vi "Set DDC Mode.vi"(0 "fpga refnum":refnum<k20>, 5 "DDC Enabled":bool, 7 "IQ Enabled":bool, 9 "DDC Frequency Shift (Hz)":dbl, 11 "error in (no error)":errorcluster) -> (4 "fpga refnum out":refnum<k20>, 8 "sample rate":dbl, 15 "error out":errorcluster)   [LabVIEW 2018, in "GettingStarted_5785_Host.lvlib"]
uses:
  GettingStarted_5785_Host.lvlib
  <instrlib>/FlexRIO/API/Host/v1/NI FlexRIO/API/Get Property Reference - Fpga Small.vi
  <resource>/objmgr/niflexrioapiStream.rc
  <instrlib>/FlexRIO/API/Host/v1/NI FlexRIO API v1.lvlib
  <resource>/objmgr/niflexrioapiChannel.rc
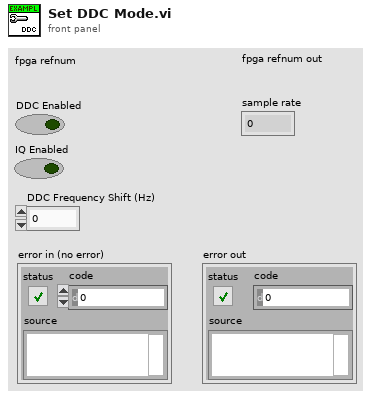
[diagram p1: front panel]
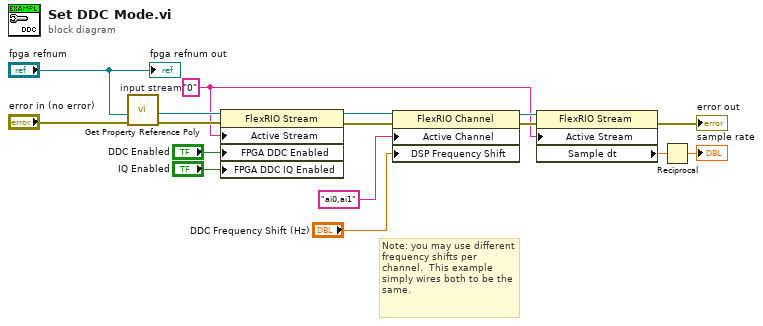
[diagram p0: block diagram]
diagram:
  w1 = "0"  # input stream
  # "Note: you may use different frequency shifts per channel.  This example simply wires both to be the same."
  n1 = call-poly <instrlib>:"Get Property Reference Poly.vi"("error in (no error)"="error in (no error)", "fpga interface in"="fpga refnum") -> ("error out"=w14:errorcluster, "property reference"=w13:refnum<k20>)  [unwired: 4 in, 1 out]
  n2 = property class="FlexRIO Stream"(reference=w13, error in=w14, "Active Stream"=w1, "FPGA DDC Enabled"="DDC Enabled", "FPGA DDC IQ Enabled"="IQ Enabled") -> (reference out=w9:refnum<k20>, error out=w8:errorcluster)
  n3 = property class="FlexRIO Channel"(reference=w9, error in=w8, "Active Channel"="ai0,ai1" ("Active Stream"), "DSP Frequency Shift"="DDC Frequency Shift (Hz)") -> (reference out=w5:refnum<k20>, error out=w6:errorcluster)
  n4 = property class="FlexRIO Stream"(reference=w5, error in=w6, "Active Stream"=w1) -> (error out=→"error out":errorcluster, "Sample dt"=w3:dbl)  [unwired: 1 out]
  n5 = Reciprocal(x=w3) -> (1/x=→"sample rate":dbl)
  "fpga refnum out" <- "fpga refnum"
